vi "zad2.vi"(8 "error in (no error)":errorcluster, 10 "Numeric 2":dbl, 11 "Numeric":dbl) -> (0 "error out":errorcluster, 3 "Array":dbl[][](array[numeric]))   [LabVIEW 2017]
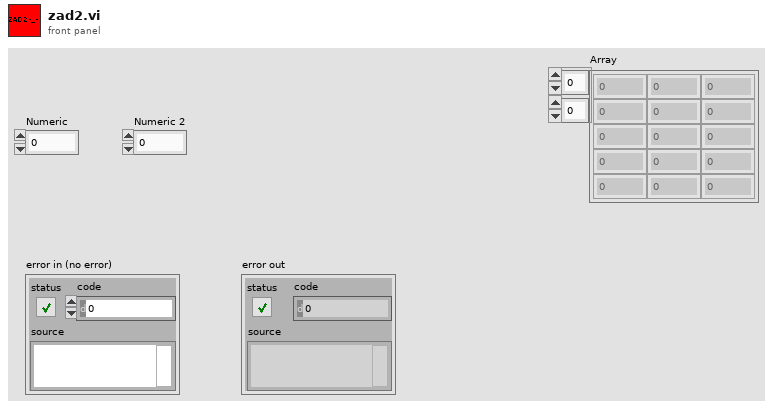
[diagram p1: front panel]
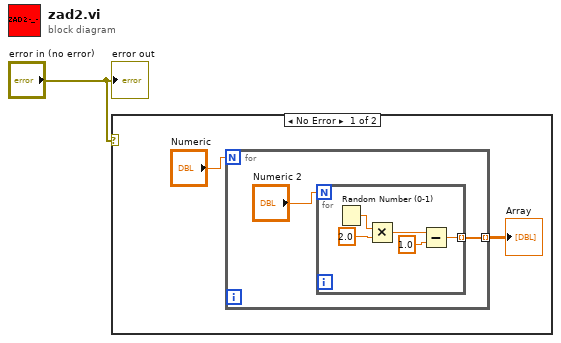
[diagram p0: block diagram]
diagram:
  n1 = case shown="No Error" "error in (no error)" {
    frame No Error {
      n2 = for {
        N: "Numeric" -> [_]
        tunnel: [w4] -> w3 mode=indexing
        n3 = for {
          N: "Numeric 2" -> [_]
          tunnel: [w6] -> w4 mode=indexing
          n4 = Random Number (0-1)() -> (number: 0 to 1=w9:dbl)
          n5 = Multiply(x=w9, y=2.0 ("Numeric 3")) -> (x*y=w7:dbl)
          n6 = Subtract(x=w7, y=1.0 ("Numeric 3")) -> (x-y=w6:dbl)
        }
      }
      "Array" <- w3
    }
    frame Error {
    }
  }
  "error out" <- "error in (no error)"
